vi "GetRegion.vi"(2 "IntGraph REF":refnum<vi>, 5 "Y Width (PX)":dbl, 9 "X Width (PX)":dbl, 13 "Action":u16(ring) items=["Set Region", "Get Region"]) -> (8 "Region Out":sgl[][](array[numeric]))   [LabVIEW 2014]
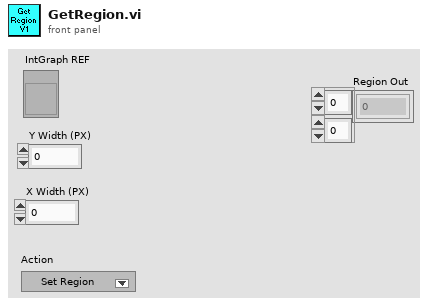
[diagram p1: front panel]
types:
  T1 = typedef "LVRectTypeDef.ctl" = cluster{"Left":i16, "Top":i16, "Right":i16, "Bottom":i16}
  T2 = typedef "LVPoint32TypeDef.ctl" = cluster{"Horizontal":i32, "Vertical":i32}
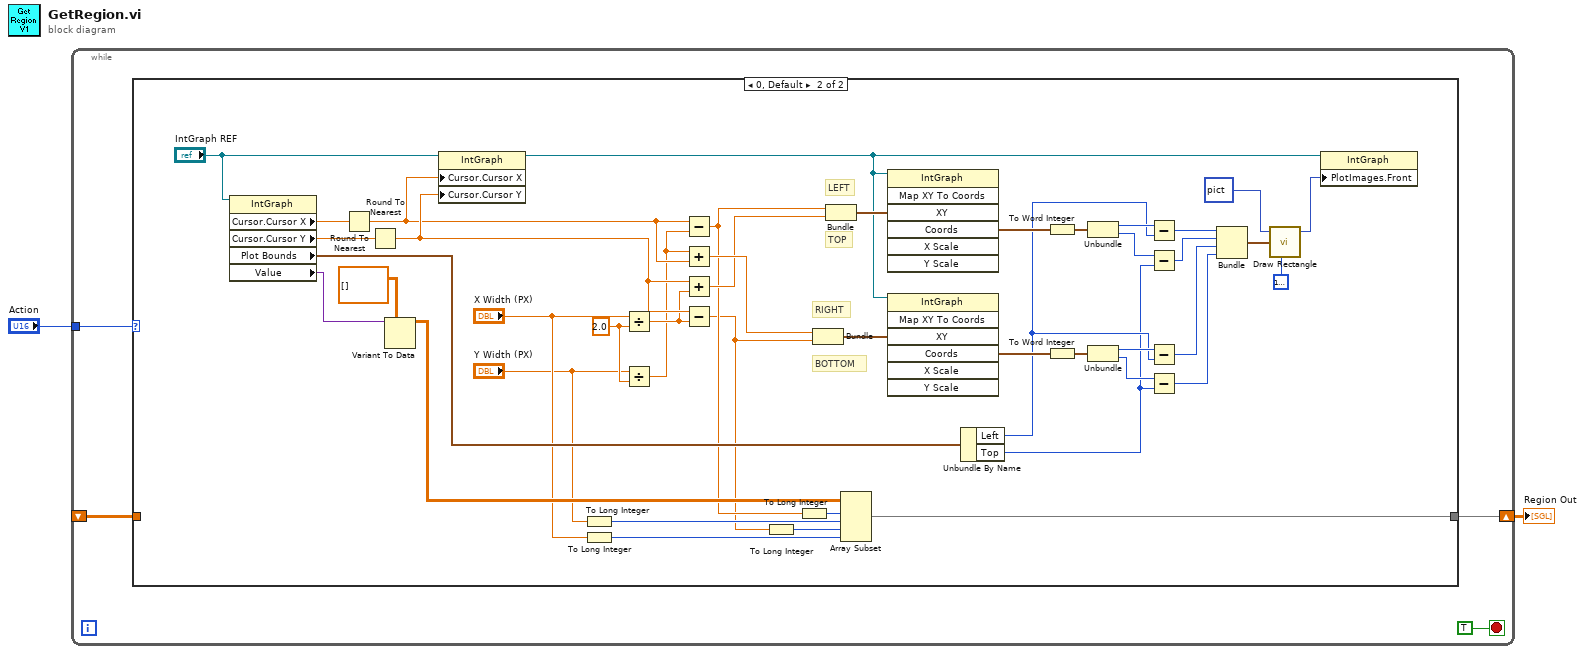
[diagram p0: block diagram]
diagram:
  n1 = while {
    shift-right: [w4] -> w1
    shift-left: _ -> [w3]
    tunnel: "Action" -> [w6]
    stop <- TRUE stop-if-true
    n2 = case shown="0, Default" w6 {
      tunnel: [w7 w8] -> w4
      tunnel: w3 -> [w7 _]
      frame 1 {
      }
      frame 0, Default {
        w51 = 2.0 ("y")
        # "BOTTOM"
        # "RIGHT"
        # "TOP"
        # "LEFT"
        n3 = property class="IntGraph"(reference="IntGraph REF") -> ("Cursor.Cursor X"=w50:dbl, "Cursor.Cursor Y"=w49:dbl, "Plot Bounds"=w19:T1, "Value"=w24:variant)  [unwired: 1 in, 2 out]
        n4 = Round To Nearest(number=w50) -> (nearest integer value=w45:dbl)
        n5 = Round To Nearest(number=w49) -> (nearest integer value=w48:dbl)
        n6 = Variant To Data(type=sgl[][] [], Variant=w24) -> (data=w20:sgl[][])  [unwired: 1 in, 1 out]
        n7 = property class="IntGraph"(reference="IntGraph REF", "Cursor.Cursor X"=w45, "Cursor.Cursor Y"=w48) -> (reference out=w11:refnum<vi>)  [unwired: 1 in, 1 out]
        n8 = To Long Integer(number="Y Width (PX)") -> (32bit integer=w16:i32)
        n9 = To Long Integer(number="X Width (PX)") -> (32bit integer=w15:i32)
        n10 = Divide(x="X Width (PX)", y=w51) -> (x/y=w26:dbl)
        n11 = Divide(x="Y Width (PX)", y=w51) -> (x/y=w25:dbl)
        n12 = Subtract(x=w45, y=w25) -> (x-y=w14:dbl)
        n13 = Add(x=w25, y=w45) -> (x+y=w22:dbl)
        n14 = Add(x=w48, y=w26) -> (x+y=w21:dbl)
        n15 = Subtract(x=w48, y=w26) -> (x-y=w13:dbl)
        n16 = To Long Integer(number=w13) -> (32bit integer=w10:i32)
        n17 = To Long Integer(number=w14) -> (32bit integer=w9:i32)
        n18 = Bundle(w22, w13) -> (w41:cluster{dbl, dbl})  [unwired: 1 in]
        n19 = Bundle(w14, w21) -> (w42:cluster{dbl, dbl})  [unwired: 1 in]
        n20 = Array Subset(array=w20, index (row)=w9, length (row)=w16, index (col)=w10, length (col)=w15) -> (w8:sgl[][])
        n21 = invoke class="IntGraph" method="Map XY To Coords"(reference=w11, "XY"=w42) -> ("Coords"=w44:T2)  [unwired: 5 in, 6 out]
        n22 = invoke class="IntGraph" method="Map XY To Coords"(reference=w11, "XY"=w41) -> ("Coords"=w43:T2)  [unwired: 5 in, 6 out]
        n23 = Unbundle By Name(w19) -> ("Left"=w28:i16, "Top"=w27:i16)
        n24 = To Word Integer(number=w44) -> (16bit integer=w40:cluster{"Horizontal":i16, "Vertical":i16})
        n25 = To Word Integer(number=w43) -> (16bit integer=w39:cluster{"Horizontal":i16, "Vertical":i16})
        n26 = Unbundle(w40) -> ("Horizontal"=w36:i16, "Vertical"=w34:i16)
        n27 = Unbundle(w39) -> ("Horizontal"=w32:i16, "Vertical"=w30:i16)
        n28 = Subtract(x=w36, y=w28) -> (x-y=w35:i16)
        n29 = Subtract(x=w34, y=w27) -> (x-y=w33:i16)
        n30 = Subtract(x=w32, y=w28) -> (x-y=w31:i16)
        n31 = Subtract(x=w30, y=w27) -> (x-y=w29:i16)
        n32 = Bundle(w35, w33, w31, w29) -> (w38:cluster{i16, i16, i16, i16})  [unwired: 1 in]
        n33 = call <vilib>:"Draw Rectangle.vi"("picture"=picture data[5B], "rect"=w38, "color(black)"=u32 16777226) -> ("new picture"=w46:picture)  [unwired: 6 in]
        n34 = property class="IntGraph"(reference=w11, "PlotImages.Front"=w46) -> ()  [unwired: 1 in, 2 out]
      }
    }
  }
  "Region Out" <- w1
